vi "UpdateViconIMUParam.vi"(8 "error in (no error)":errorcluster) -> (0 "error out":errorcluster)   [LabVIEW 2015]
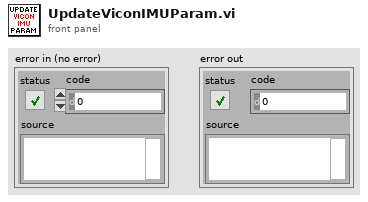
[diagram p1: front panel]
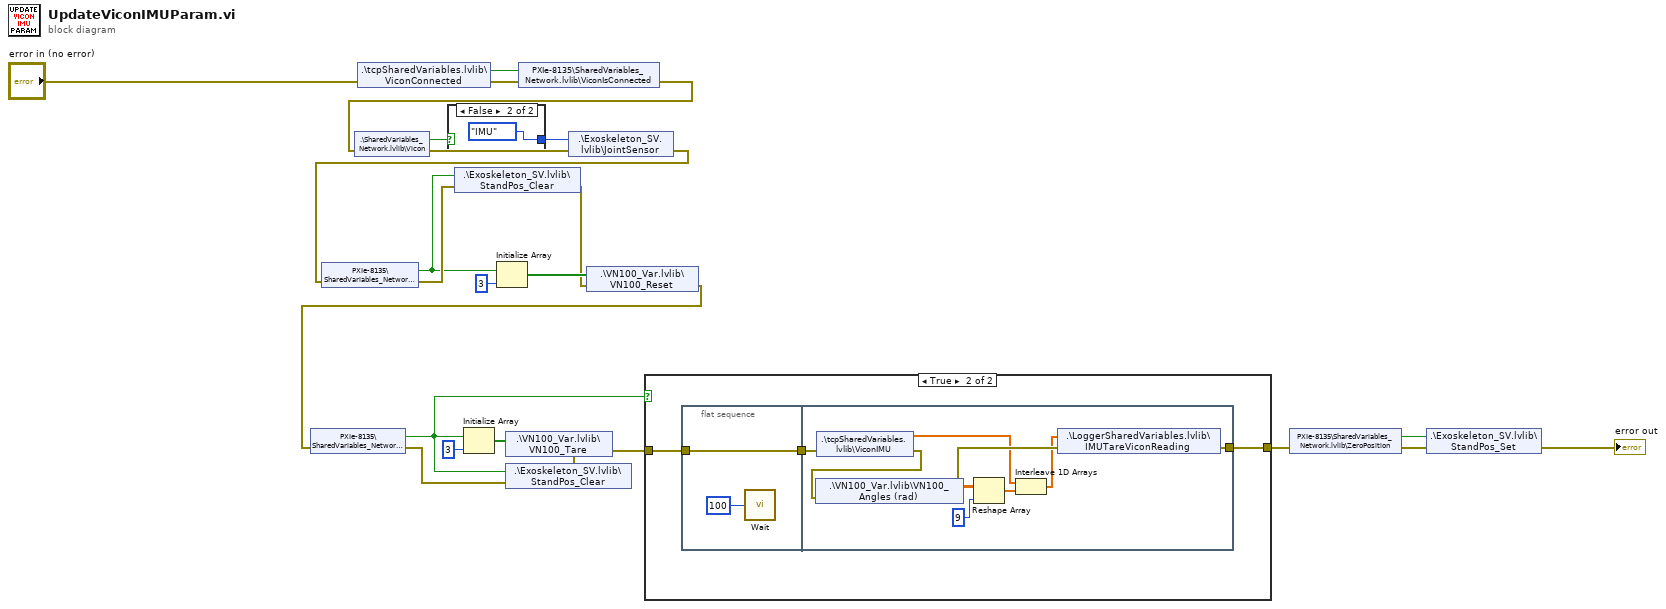
[diagram p0: block diagram]
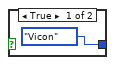
[diagram p3: hidden frame]
diagram:
  n1 = shared-variable ".\\tcpSharedVariables.lvlib\\ViconConnected"(error in="error in (no error)") -> (w18:bool, error out=w17:errorcluster)
  n2 = shared-variable "PXIe-8135\\SharedVariables_Network.lvlib\\ViconIsConnected"(w18, error in=w17) -> (error out=w19:errorcluster)
  n3 = shared-variable ".\\SharedVariables_Network.lvlib\\Vicon"(error in=w19) -> (w21:bool, error out=w20:errorcluster)
  n4 = case shown="False" w21 {
    tunnel: [enum16{"IMU", "Vicon"}."Vicon" ("JointSensor") enum16{"IMU", "Vicon"}."IMU" ("JointSensor")] -> w22
    frame True {
    }
    frame False {
    }
  }
  n5 = shared-variable ".\\Exoskeleton_SV.lvlib\\JointSensor"(w22, error in=w20) -> (error out=w23:errorcluster)
  n6 = shared-variable "PXIe-8135\\SharedVariables_Network.lvlib\\IMU_reset"(error in=w23) -> (w11:bool, error out=w13:errorcluster)
  n7 = shared-variable ".\\Exoskeleton_SV.lvlib\\StandPos_Clear"(w11, error in=w13) -> (error out=w12:errorcluster)
  n8 = Initialize Array(w11, 3 ("dimension size")) -> (w15:bool[])
  n9 = shared-variable ".\\VN100_Var.lvlib\\VN100_Reset"(w15, error in=w12) -> (error out=w16:errorcluster)
  n10 = shared-variable "PXIe-8135\\SharedVariables_Network.lvlib\\IMU_Tare"(error in=w16) -> (w2:bool, error out=w10:errorcluster)
  n11 = Initialize Array(w2, 3 ("dimension size")) -> (w8:bool[])
  n12 = shared-variable ".\\Exoskeleton_SV.lvlib\\StandPos_Clear"(w2, error in=w10) -> (error out=w4:errorcluster)
  n13 = shared-variable ".\\VN100_Var.lvlib\\VN100_Tare"(w8, error in=w4) -> (error out=w3:errorcluster)
  n14 = case shown="True" w2 {
    tunnel: w3 -> [w27 w30]
    tunnel: [w27 w29] -> w1
    frame False {
    }
    frame True {
      n15 = flat-sequence {
        tunnel: w30 -> [w32]
        tunnel: [w32] -> w28
        tunnel: [w33] -> w29
        tunnel: w28 -> [w41]
        frame #0 {
          n16 = call "Wait"("Count(mSec)"=u32 100 ("milliseconds to wait")) -> ()  [unwired: 1 out]
        }
        frame #1 {
          n17 = shared-variable ".\\tcpSharedVariables.lvlib\\ViconIMU"(error in=w41) -> (w35:dbl[], error out=w40:errorcluster)
          n18 = shared-variable ".\\VN100_Var.lvlib\\VN100_Angles (rad)"(error in=w40) -> (w39:dbl[][], error out=w37:errorcluster)
          n19 = Reshape Array(w39, 9 ("dimension size")) -> (w36:dbl[])
          n20 = Interleave 1D Arrays(w35, w36) -> (w34:dbl[])
          n21 = shared-variable ".\\LoggerSharedVariables.lvlib\\IMUTareViconReading"(w34, error in=w37) -> (error out=w33:errorcluster)
        }
      }
    }
  }
  n22 = shared-variable "PXIe-8135\\SharedVariables_Network.lvlib\\ZeroPosition"(error in=w1) -> (w7:bool, error out=w6:errorcluster)
  n23 = shared-variable ".\\Exoskeleton_SV.lvlib\\StandPos_Set"(w7, error in=w6) -> (error out=→"error out":errorcluster)
